vi "Initialize Input Offset.vi"(8 "error in (no error)":errorcluster, 11 "Instrument.DAQ":refnum<class "Instrument.DAQ.lvclass">) -> (0 "error out":errorcluster, 3 "Instrument.DAQ out":refnum<class "Instrument.DAQ.lvclass">)   [LabVIEW 2019, in "Instrument.DAQ.lvclass"]
uses:
  Instrument.DAQ.lvclass
  Instrument.DAQ.lvclass/Instrument.DAQ.ctl
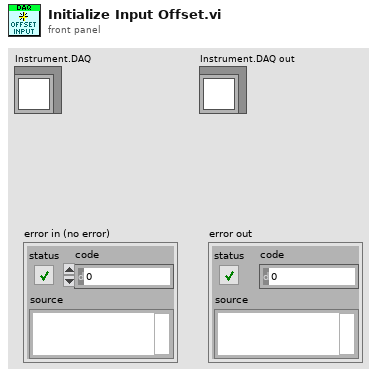
[diagram p1: front panel]
types:
  T1 = typedef "Instrument.DAQ.lvclass/Channel.Gain--Cluster--Array.ctl" = T2[]
  T2 = typedef "Instrument.DAQ.lvclass/Channel.Gain--Cluster.ctl" = cluster{"Channel":string, "Gain":dbl}
  T3 = typedef "Instrument.DAQ.lvclass/DAQ.Config.AO--Cluster--Array.ctl" = T4[]
  T4 = typedef "Instrument.DAQ.lvclass/DAQ.Config.AO--Cluster.ctl" = cluster{"Channels":tag, "Range":T5, "output terminal configuration":i32, "Type":T6}
  T5 = typedef "Instrument.DAQ.lvclass/DAQ.Config.AO.Range--enum.ctl" = enum16{"±0.1", "±1.0", "±10.0"}
  T6 = typedef "Instrument.DAQ.lvclass/DAQ.Type--enum.ctl" = enum16{"None", "USB-4431", "PXI-446x"}
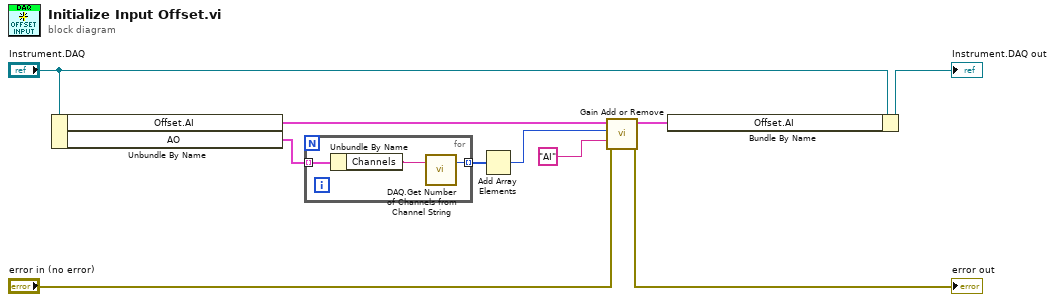
[diagram p0: block diagram]
diagram:
  n1 = Unbundle By Name("Instrument.DAQ") -> ("Offset.AI"=w7:T1, "AO"=w1:T3)
  n2 = for {
    tunnel: w1 -> [w13] mode=indexing
    tunnel: [w11] -> w10 mode=indexing
    n3 = Unbundle By Name(w13) -> ("Channels"=w12:tag)
    n4 = call "DAQ.Get Number of Channels from Channel String.vi"("Channels String"=w12) -> ("# channels"=w11:i32)  [unwired: 2 in]
  }
  n5 = Add Array Elements(numeric array=w10) -> (sum=w5:i32)
  n6 = call "Gain Add or Remove.vi"("error in (no error)"="error in (no error)", "Name Prefix"="AI", "Size"=w5, "Channel Gain"=w7) -> ("error out"=→"error out":errorcluster, "Channel Gain out"=w2:T1)  [unwired: 6 in]
  n7 = Bundle By Name(cluster="Instrument.DAQ", "Offset.AI"=w2) -> (→"Instrument.DAQ out":refnum<class "Instrument.DAQ.lvclass">)
